vi "Get Localized Text.vi"(7 "Text Type":enum16{"Status", "Title", "Controls"}(ring), 9 "Text Index":i32, 10 "Force Index":bool, 11 "Data In":T1 {"Language" items=["English", "Español", "Português"]}) -> (1 "Localized Text":string, 3 "Data Out":T1 {"Language" items=["English", "Español", "Português"]})   [LabVIEW 2017]
uses:
  Controls/HID Data.ctl
  <vilib>/userdefined/High Color/IMAQdx.ctl
  <vilib>/vision/Image Controls.llb/IMAQ Image.ctl
  Controls/HID State.ctl
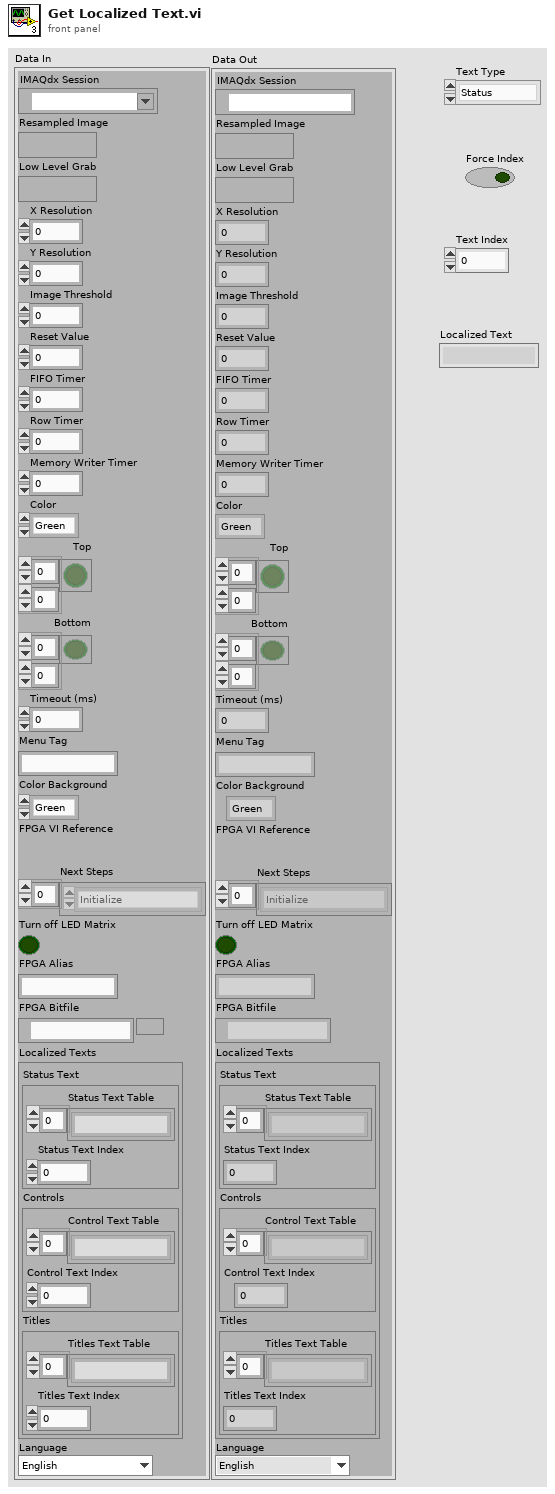
[diagram p1: front panel]
types:
  T1 = typedef "HID Data.ctl" = cluster{"IMAQdx Session":T2, "Resampled Image":T3, "Low Level Grab":T3, "X Resolution":i32, "Y Resolution":i32, "Image Threshold":u8, "Reset Value":i32, "FIFO Timer":u16, "Row Timer":u32, "Memory Writer Timer":u8, "Color":enum16{"Green", "Blue", "Red", "White", "Pink", "Yellow", "Turquoise", "Black"}, "Top":bool[][], "Bottom":bool[][], "Timeout (ms)":i32, "Menu Tag":string, "Color Background":enum16{"Green", "Blue", "Red", "White", "Pink", "Yellow", "Turquoise", "Black"}, "FPGA VI Reference":refnum<k20>, "Next Steps":T4[], "Turn off LED Matrix":bool, "FPGA Alias":string, "FPGA Bitfile":path, "Localized Texts":cluster{"Status Text":cluster{"Status Text Table":string[], "Status Text Index":i32}, "Controls":cluster{"Control Text Table":string[], "Control Text Index":i32}, "Titles":cluster{"Titles Text Table":string[], "Titles Text Index":i32}}, "Language":u16}
  T2 = typedef "IMAQdx.ctl" = refnum<k21>
  T3 = typedef "IMAQ Image.ctl" = refnum<image>
  T4 = typedef "HID State.ctl" = enum16{"Initialize", "Set FPGA Parametes", "Set Camera Parameters", "Set LED Matrix Parameters", "Initialize FPGA Interface", "Initialize Camera", "Start FPGA VI", "Start Camera", "Wait for Event", "Update UI", "Acquire", "Process Image", "Get Boolean Arrays", "Send to FPGA", "Menu Pop-Up", "Menu Actions", "Handle Errors", "Close Camera", "Close FPGA", "Stop", "Exit"}
  T5 = cluster{"Titles Text Table":string[], "Titles Text Index":i32}
  T6 = cluster{"Control Text Table":string[], "Control Text Index":i32}
  T7 = cluster{"Status Text Table":string[], "Status Text Index":i32}
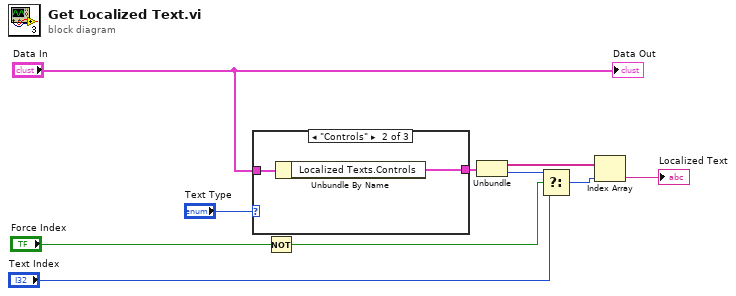
[diagram p0: block diagram]
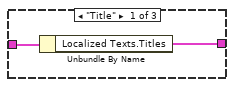
[diagram p2: hidden frame]
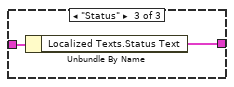
[diagram p3: hidden frame]
diagram:
  n1 = case shown="\"Controls\"" "Text Type" {
    tunnel: "Data In" -> [w12 w14 w16]
    tunnel: [w11 w13 w15] -> w9
    frame "Title" {
      n2 = Unbundle By Name(w12) -> ("Localized Texts.Titles"=w11:T5)
    }
    frame "Controls" {
      n3 = Unbundle By Name(w14) -> ("Localized Texts.Controls"=w13:T6)
    }
    frame "Status" {
      n4 = Unbundle By Name(w16) -> ("Localized Texts.Status Text"=w15:T7)
    }
  }
  n5 = Not(x="Force Index") -> (.not. x?=w1:bool)
  n6 = Unbundle(w9) -> ("Status Text Table"=w8:string[], "Status Text Index"=w5:i32)
  n7 = Select(t=w5, s=w1, f="Text Index") -> (s? t:f=w4:i32)
  n8 = Index Array(array=w8, index=w4) -> (element=→"Localized Text":string)
  "Data Out" <- "Data In"
